vi "Grubber Controller.vi"(8 "error in":errorcluster) -> ()   [LabVIEW 2017]
doc: "This VI executes continuously carrying out the current operation and responding to updates or new operations. It will often contain the timing or control code that is difficult to place directly in TeleOp. This VI generally opens all sensors and motors and isolates the rest of the robot code from knowing how the operations are carried out."
uses:
  <vilib>/Rock Robotics/WPI/Framework/Completion Status.ctl
  Grubber Setpoints.ctl
  Grubber Operations.ctl
  <vilib>/Rock Robotics/SystemInterfaces/DIO/FPGA_DIOPWMChannel.ctl
  <vilib>/Rock Robotics/WPI/SafetyOutput/WPI_SafetyOutputConfigMenu.ctl
  <vilib>/Rock Robotics/WPI/MotorControl/WPI_MotorControlOpen SPARK.vi
  <vilib>/Rock Robotics/Network Tables/NT Write Number.vi
panel:
  in  "Interactive Values":T1
  out "Current\nCmd":string
  in  "Buttons":cluster{"Execute Cmd":bool, "Abort Cmd":bool}
  out "Command Timing":cluster{"Start Time (ms)":u32, "Iterations":i32}
  out "Status":T3
  # "Tip: It may be helpful to observe inputs and sensor values.\nYou may also want to display tuning or debugging controls."
  # "Interactive Command: You may fill in the settings for a command\nand schedule it with the Execute button. You can observe and abort\nany command while fine tuning the code for the controller."
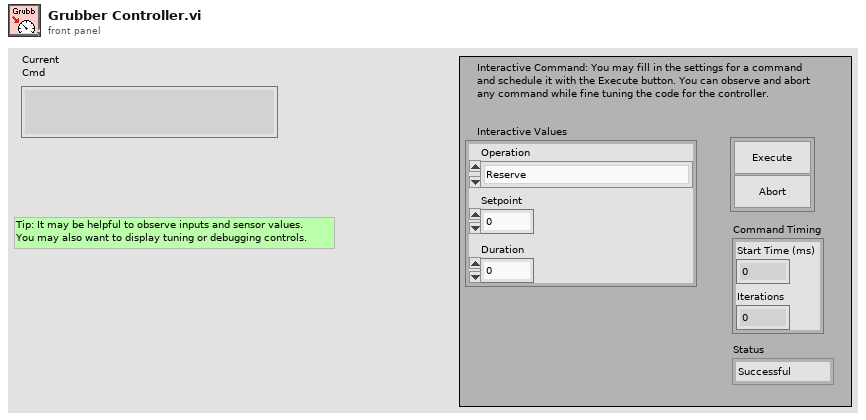
[diagram p1: front panel]
types:
  T1 = typedef "Grubber Setpoints.ctl" = cluster{"Operation":T2, "Setpoint":dbl, "Duration":dbl}
  T2 = typedef "Grubber Operations.ctl" = enum16{"Reserve", "Read Current", "Immediate", "Grab for Time", "Grab", "Release"}
  T3 = typedef "Completion Status.ctl" = enum16{"Successful", "Aborted", "Incomplete"}
  T4 = typedef "WPI_SafetyOutputConfigMenu.ctl" = enum16{"Enable", "Disable"}
  T5 = typedef "FPGA_DIOPWMChannel.ctl" = enum8{"PWM 0", "PWM 1", "PWM 2", "PWM 3", "PWM 4", "PWM 5", "PWM 6", "PWM 7", "PWM 8", "PWM 9", "PWM MXP 0", "PWM MXP 1", "PWM MXP 2", "PWM MXP 3", "PWM MXP 4", "PWM MXP 5", "PWM MXP 6", "PWM MXP 7", "PWM MXP 8", "PWM MXP 9", "Invalid"}
  T6 = typedef "WPI_MotorControlDeviceRef.ctl" = cluster{"DeviceStatus":errorcluster, "Type":T7, "PWM":cluster{"PWM Channel":T5, "DeadBand":T8}, "CAN":cluster{"Device Number":u8, "SetOutput VI Ref":variant, "GetOutput VI Ref":variant, "Enable VI Ref":variant, "Disable VI Ref":variant, "Data":variant}, "Invert":bool, "DIO PWM":cluster{"PWM \"Enable\" Channel":T5, "DIOChannel":T9, "PWM Rate":dbl}}
  T7 = typedef "WPI_MotorControlType.ctl" = enum16{"PWM", "CAN", "DIO PWM"}
  T8 = typedef "WPI_PWMDeadband.ctl" = cluster{"Name":string, "maxPositivePwm":i32, "minPositivePwm":i32, "centerPwm":i32, "maxNegativePwm":i32, "minNegativePwm":i32, "angularRange":u16}
  T9 = typedef "FPGA_DIOChannel.ctl" = enum8{"DIO 0", "DIO 1", "DIO 2", "DIO 3", "DIO 4", "DIO 5", "DIO 6", "DIO 7", "DIO 8", "DIO 9", "DIO MXP 0", "DIO MXP 1", "DIO MXP 2", "DIO MXP 3", "DIO MXP 4", "DIO MXP 5", "DIO MXP 6", "DIO MXP 7", "DIO MXP 8", "DIO MXP 9", "DIO MXP 10", "DIO MXP 11", "DIO MXP 12", "DIO MXP 13", "DIO MXP 14", "DIO MXP 15", "SPI Port CS1", "SPI Port CS2", "SPI Port CS3", "SPI Port MISO", "SPI Port MOSI", "Invalid"}
  T10 = typedef "Command Status Info.ctl" = cluster{"Name":string, "Status":T3, "notifier out":T11}
  T11 = typedef "Completion Notifier.ctl" = refnum<notifier>
  T12 = cluster{"Current Command":T1, "Command Timing":cluster{"Start Time (ms)":u32, "Iterations":i32}, "Command Arguments":cluster{"Command Info":T10, "Description":string, "Default Command":T1, "queue out":refnum<queue>, "Subsystem Name":string}}
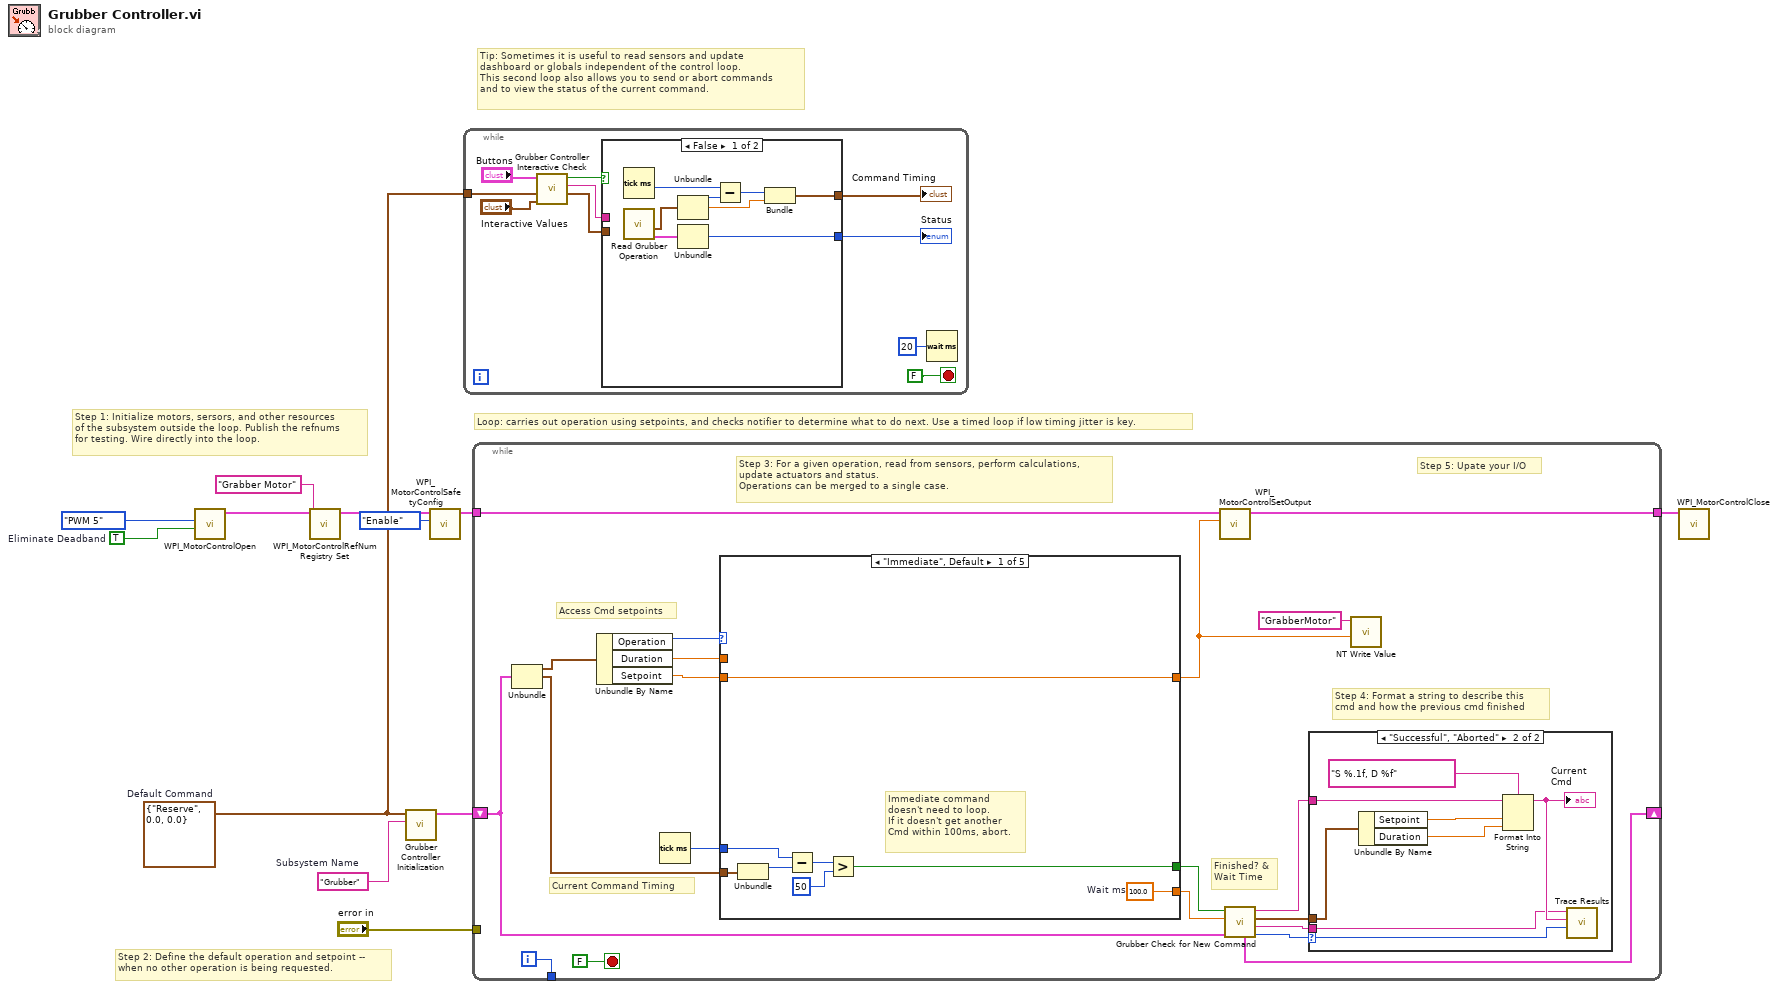
[diagram p0: block diagram]
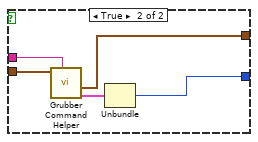
[diagram p2: hidden frame]
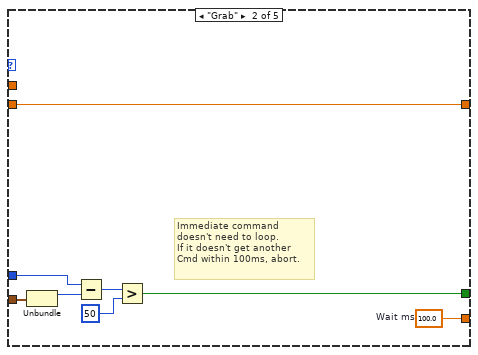
[diagram p4: hidden frame]
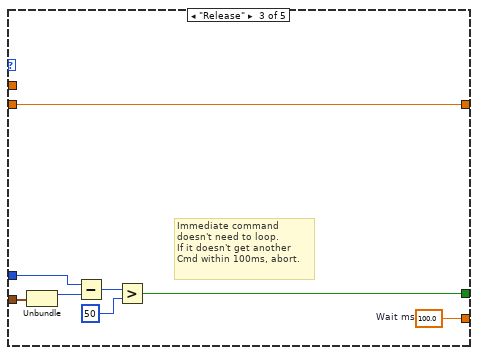
[diagram p5: hidden frame]
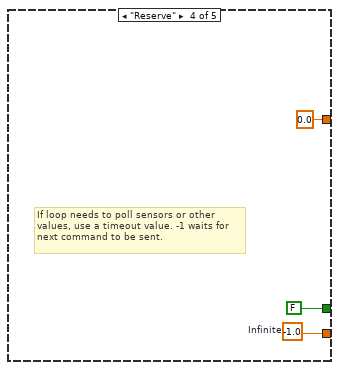
[diagram p6: hidden frame]
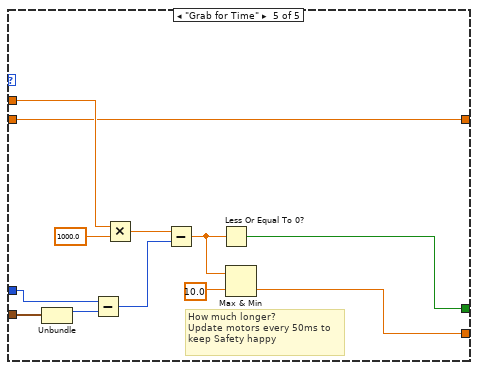
[diagram p7: hidden frame]
diagram:
  w7 = TRUE  # Eliminate Deadband
  w9 = T1 {"Operation"=enum."Reserve", "Setpoint"=0.0, "Duration"=0.0}  # Default Command
  w10 = "Grubber"  # Subsystem Name
  # "Tip: Sometimes it is useful to read sensors and update\ndashboard or globals independent of the control loop.\nThis second loop also allows you to send or abort commands\nand to view the status of the current command."
  # "Step 2: Define the default operation and setpoint --\nwhen no other operation is being requested."
  # "Step 1: Initialize motors, sersors, and other resources\nof the subsystem outside the loop. Publish the refnums\nfor testing. Wire directly into the loop."
  # "Loop: carries out operation using setpoints, and checks notifier to determine what to do next. Use a timed loop if low timing jitter is key."
  n1 = call-poly <vilib>:"WPI_MotorControlOpen.vi"("Eliminate Deadband"=w7, "PWM Channel"=FPGA_DIOPWMChannel."PWM 5") -> ("MotorControlDeviceRef"=w6:T6)  [unwired: 8 in, 1 out]
  n2 = call <vilib>:"WPI_MotorControlRefNum Registry Set.vi"("refnum name"="Grabber Motor", "MotorControlDevRef"=w6) -> ("MotorControlDevRef"=w5:T6)  [unwired: 8 in, 1 out]
  n3 = call "Grubber Controller Initialization.vi"("Subsystem Name"=w10, "Default Command"=w9) -> ("Current Command"=w11:T12)  [unwired: 9 in]
  n4 = call <vilib>:"WPI_MotorControlSafetyConfig.vi"("mode"=WPI_SafetyOutputConfigMenu."Enable", "MotorControlDevRef"=w5) -> ("MotorControlDevRef"=w3:T6)  [unwired: 8 in, 1 out]
  n5 = while {
    tunnel: w9 -> [w19]
    stop <- FALSE stop-if-true
    n6 = call "Grubber Controller Interactive Check.vi"("Interactive Command in"="Interactive Values", "Default Command"=w19, "Buttons"="Buttons") -> ("Interactive Command out"=w16:T1, "Trace String"=w17:string, "Schedule"=w18:bool)  [unwired: 6 in]
    n7 = case shown="False" w18 {
      tunnel: [w30 w35] -> w15
      tunnel: w16 -> [_ w33]
      tunnel: [w26 w31] -> w14
      tunnel: w17 -> [_ w34]
      frame False {
        n8 = Tick Count (ms)() -> (millisecond timer value=w25:u32)
        n9 = call "Read Grubber Operation.vi"() -> ("Command Info"=w23:T10, "SubSystem Data"=w24:T1)  [unwired: 9 in, 1 out]
        n10 = Unbundle(w24) -> ("Operation"=w29:T2, "Setpoint"=w27:dbl)  [unwired: 1 out]
        n11 = Unbundle(w23) -> ("Status"=w30:T3)  [unwired: 2 out]
        n12 = Subtract(x=w25, y=w29) -> (x-y=w28:u32)
        n13 = Bundle(w28, "Setpoint"=w27) -> (w26:cluster{u32, "Setpoint":dbl})  [unwired: 1 in]
      }
      frame True {
        n14 = call "Grubber Command Helper.vi"("Description"=w34, "SubSystem Data"=w33) -> ("Command Info Out"=w32:T10, "Command Timing"=w31:cluster{"Start Time (ms)":u32, "Iterations":i32})  [unwired: 7 in, 1 out]
        n15 = Unbundle(w32) -> ("Status"=w35:T3)  [unwired: 2 out]
      }
    }
    "Status" <- w15
    "Command Timing" <- w14
    n16 = Wait (ms)(milliseconds to wait=u32 20) -> ()  [unwired: 1 out]
  }
  n17 = while {
    shift-right: [w47] -> _
    shift-left: w11 -> [w40]
    tunnel: [w54] -> _
    tunnel: "error in" -> [_]
    tunnel: w3 -> [w39]
    tunnel: [w37] -> w2
    i -> [w54]
    stop <- FALSE stop-if-true
    # "Step 5: Upate your I/O"
    # "Step 4: Format a string to describe this\ncmd and how the previous cmd finished"
    # "Current Command Timing"
    # "Access Cmd setpoints"
    # "Finished? &\nWait Time"
    # "Step 3: For a given operation, read from sensors, perform calculations,\nupdate actuators and status.\nOperations can be merged to a single case."
    n18 = Unbundle(w40) -> ("Current Command"=w53:T1, "Command Timing"=w49:cluster{"Start Time (ms)":u32, "Iterations":i32})  [unwired: 1 out]
    n19 = Unbundle By Name(w53) -> ("Operation"=w52:T2, "Duration"=w51:dbl, "Setpoint"=w48:dbl)
    n20 = Tick Count (ms)() -> (millisecond timer value=w50:u32)
    n21 = case shown="\"Immediate\", Default" w52 {
      tunnel: [w71 w79 w87 w90 w92] -> w45
      tunnel: [w65 w73 w81 FALSE ("ignore previous (F)") w93] -> w46
      tunnel: w49 -> [w67 w75 w83 _ w96]
      tunnel: w51 -> [_ _ _ _ w94]
      tunnel: w50 -> [w66 w74 w82 _ w95]
      tunnel: w48 -> [w64 w72 w80 _ w91]
      tunnel: [w64 w72 w80 0.0 ("Setpoint") w91] -> w36
      frame "Immediate", Default {
        w71 = 100.0  # Wait ms
        # "Immediate command\ndoesn't need to loop.\nIf it doesn't get another\nCmd within 100ms, abort."
        n22 = Unbundle(w67) -> ("Start Time (ms)"=w70:u32)  [unwired: 1 out]
        n23 = Subtract(x=w66, y=w70) -> (x-y=w69:u32)
        n24 = Greater?(x=w69, y=u8 50 ("Left Motor")) -> (0:w65:bool)
      }
      frame "Grab" {
        w79 = 100.0  # Wait ms
        # "Immediate command\ndoesn't need to loop.\nIf it doesn't get another\nCmd within 100ms, abort."
        n25 = Unbundle(w75) -> ("Start Time (ms)"=w78:u32)  [unwired: 1 out]
        n26 = Subtract(x=w74, y=w78) -> (x-y=w77:u32)
        n27 = Greater?(x=w77, y=u8 50 ("Left Motor")) -> (0:w73:bool)
      }
      frame "Release" {
        w87 = 100.0  # Wait ms
        # "Immediate command\ndoesn't need to loop.\nIf it doesn't get another\nCmd within 100ms, abort."
        n28 = Unbundle(w83) -> ("Start Time (ms)"=w86:u32)  [unwired: 1 out]
        n29 = Subtract(x=w82, y=w86) -> (x-y=w85:u32)
        n30 = Greater?(x=w85, y=u8 50 ("Left Motor")) -> (0:w81:bool)
      }
      frame "Reserve" {
        w90 = -1.0  # Infinite
        # "If loop needs to poll sensors or other\nvalues, use a timeout value. -1 waits for\nnext command to be sent."
      }
      frame "Grab for Time" {
        # "How much longer?\nUpdate motors every 50ms to\nkeep Safety happy"
        n31 = Unbundle(w96) -> ("Start Time (ms)"=w99:u32)  [unwired: 1 out]
        n32 = Subtract(x=w95, y=w99) -> (x-y=w102:u32)
        n33 = Multiply(x=w94, y=1000.0) -> (x*y=w101:dbl)
        n34 = Subtract(x=w101, y=w102) -> (x-y=w98:dbl)
        n35 = Less Or Equal To 0?(x=w98) -> (x <= 0?=w93:bool)
        n36 = Max & Min(x=w98, y=10.0) -> (min(x,y)=w92:dbl)  [unwired: 1 out]
      }
    }
    n37 = call <vilib>:"WPI_MotorControlSetOutput.vi"("Output"=w36, "MotorControlDevRef"=w39) -> ("MotorControlDevRef"=w37:T6)  [unwired: 7 in, 2 out]
    n38 = call "Grubber Check for New Command.vi"("Current Command"=w40, "Wait time (ms)"=w45, "Finished?"=w46) -> ("Completion"=w41:T3, "Subsystem Name"=w42:string, "Current Command"=w43:T1, "Initial Trace String"=w44:string, "NextCommand"=w47:T12)  [unwired: 4 in]
    n39 = case shown="\"Successful\", \"Aborted\"" w41 {
      selector: w41 -> [_ w63]
      tunnel: w44 -> [_ w59]
      tunnel: w43 -> [_ w60]
      tunnel: w42 -> [_ w56]
      frame "Incomplete", Default {
        # "Continuing current command"
      }
      frame "Successful", "Aborted" {
        # "Report and setup for next command"
        n40 = Unbundle By Name(w60) -> ("Setpoint"=w62:dbl, "Duration"=w57:dbl)
        n41 = Format Into String(format string="S %.1f, D %f", initial string=w59, w62, w57) -> (resulting string=w58:string)  [unwired: 1 in, 1 out]
        "Current\nCmd" <- w58
        n42 = call <vilib>:"Trace Results.vi"("Status of previous command"=w63, "Description"=w58, "Subsystem"=w56) -> ()  [unwired: 9 in]
      }
    }
    n43 = call-poly <vilib>:"NT Write Value.vi"("Numeric"=w36, "Name"="GrabberMotor") -> ()  [unwired: 9 in, 1 out]
  }
  n44 = call <vilib>:"WPI_MotorControlClose.vi"("MotorControlDevRef"=w2) -> ()  [unwired: 10 in, 1 out]
